vi "Teleop.vi"(10 "Match Info":T1={"Autonomous Elapsed Seconds"=0.0, "TeleOp Elapsed Seconds"=0.0, "Disabled Elapsed Seconds"=0.0, "Visited Autonomous"=FALSE, "Visited TeleOp"=FALSE, "Visited Disabled"=FALSE, "Autonomous Settings"={"Autonomous Style"=enum."Independent", "VI Refnum"=refnum}}, 11 "Call Context":T2) -> ()   [LabVIEW 2013]
doc: "This VI is called for each TeleOp packet received from the DS where the robot is not disabled. It is often used to read from the joysticks and update I/O or to update setpoints for timed control loops. It should complete and return within 20 milliseconds or it may miss DS packets."
uses:
  <vilib>/Rock Robotics/WPI/DriverStation/WPI_DriverStationDerivedRobotMode.ctl
  <vilib>/Rock Robotics/WPI/DriverStation/WPI_DriverStationMatch Info.ctl
  Robot Global Data.vi
  <vilib>/Rock Robotics/WPI/Joystick/WPI_JoystickGetSetRefNum.vi
  <vilib>/Rock Robotics/WPI/RobotDrive/WPI_RobotDriveGetSetRefNum.vi
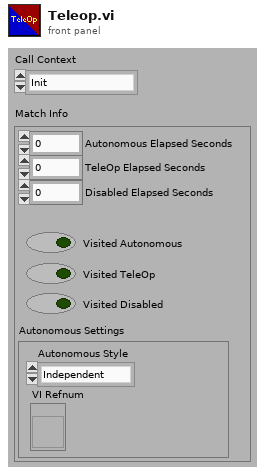
[diagram p1: front panel]
types:
  T1 = typedef "WPI_DriverStationMatch Info.ctl" = cluster{"Autonomous Elapsed Seconds":dbl, "TeleOp Elapsed Seconds":dbl, "Disabled Elapsed Seconds":dbl, "Visited Autonomous":bool, "Visited TeleOp":bool, "Visited Disabled":bool, "Autonomous Settings":cluster{"Autonomous Style":enum16{"Iterative", "Independent"}, "VI Refnum":refnum<vi>}}
  T2 = typedef "WPI_DriverStationDerivedRobotMode.ctl" = enum16{"Init", "Execute", "Stop"}
  T3 = typedef "WPI_JoystickDevRef.ctl" = cluster{"Device":T4}
  T4 = typedef "WPI_JoystickDeviceEnum.ctl" = enum16{"USB 1", "USB 2", "USB 3", "USB 4", "Kinect 1", "Kinect 2"}
  T5 = cluster{"axis 1 (x)":dbl, "axis 2 (y)":dbl, "axis 3 (throttle)":dbl, "axis 4":dbl, "axis 5":dbl, "axis 6":dbl}
  T6 = typedef "WPI_RobotDriveDevRef.ctl" = cluster{"DevStatus":errorcluster, "Motors[]":T7[], "Square Inputs":bool, "Max Output":dbl, "Isochronous":bool}
  T7 = typedef "WPI_MotorControlDeviceRef.ctl" = cluster{"DeviceStatus":errorcluster, "Type":enum16{"PWM", "CAN"}, "PWM":cluster{"Digital Module":T8, "PWM Channel":T9, "DeadBand":T10}, "CAN":cluster{"Device Number":u8, "Control Mode":T11, "Semaphore":T12, "Max Vout":dbl}, "Invert":bool, "TransformRef":T13, "InvTransformRef":T13}
  T8 = typedef "FPGA_TypedefDigitalModule.ctl" = enum16{"Digital Module 1", "Digital Module 2"}
  T9 = typedef "FPGA_DIOPWMChannel.ctl" = enum8{"PWM 1", "PWM 2", "PWM 3", "PWM 4", "PWM 5", "PWM 6", "PWM 7", "PWM 8", "PWM 9", "PWM 10", "Invalid"}
  T10 = typedef "WPI_PWMDeadband.ctl" = cluster{"Name":string, "maxPositivePwm":i32, "minPositivePwm":i32, "centerPwm":i32, "maxNegativePwm":i32, "minNegativePwm":i32, "angularRange":u16}
  T11 = typedef "WPI_CANJaguar_ControlMode.ctl" = enum8{"Percent VBus", "Current", "Speed", "Position", "Voltage"}
  T12 = typedef "Semaphore RefNum" = refnum<k1>
  T13 = typedef "WPI_PWMTransform_ConPane.ctl" = refnum<vi>
  T14 = enum16{"ToPos2", "ToPos1", "Fire", "Wait", "ESTOP", "Reset", "ToLowPower", "ToHighPower"}
  T15 = typedef "WPI_JoystickButtonState.ctl" = cluster{"Button 1":bool, "Button 2":bool, "Button 3":bool, "Button 4":bool, "Button 5":bool, "Button 6":bool, "Button 7":bool, "Button 8":bool, "Button 9":bool, "Button 10":bool, "Button 11":bool, "Button 12":bool}
  T16 = typedef "WPI_DigitalInputDevRef.ctl" = cluster{"DevStatus":errorcluster, "DIO Channel":T17, "Digital Module":T8}
  T17 = typedef "FPGA_DIOChannel.ctl" = enum8{"DIO 1", "DIO 2", "DIO 3", "DIO 4", "DIO 5", "DIO 6", "DIO 7", "DIO 8", "DIO 9", "DIO 10", "DIO 11", "DIO 12", "DIO 13", "DIO 14", "Invalid"}
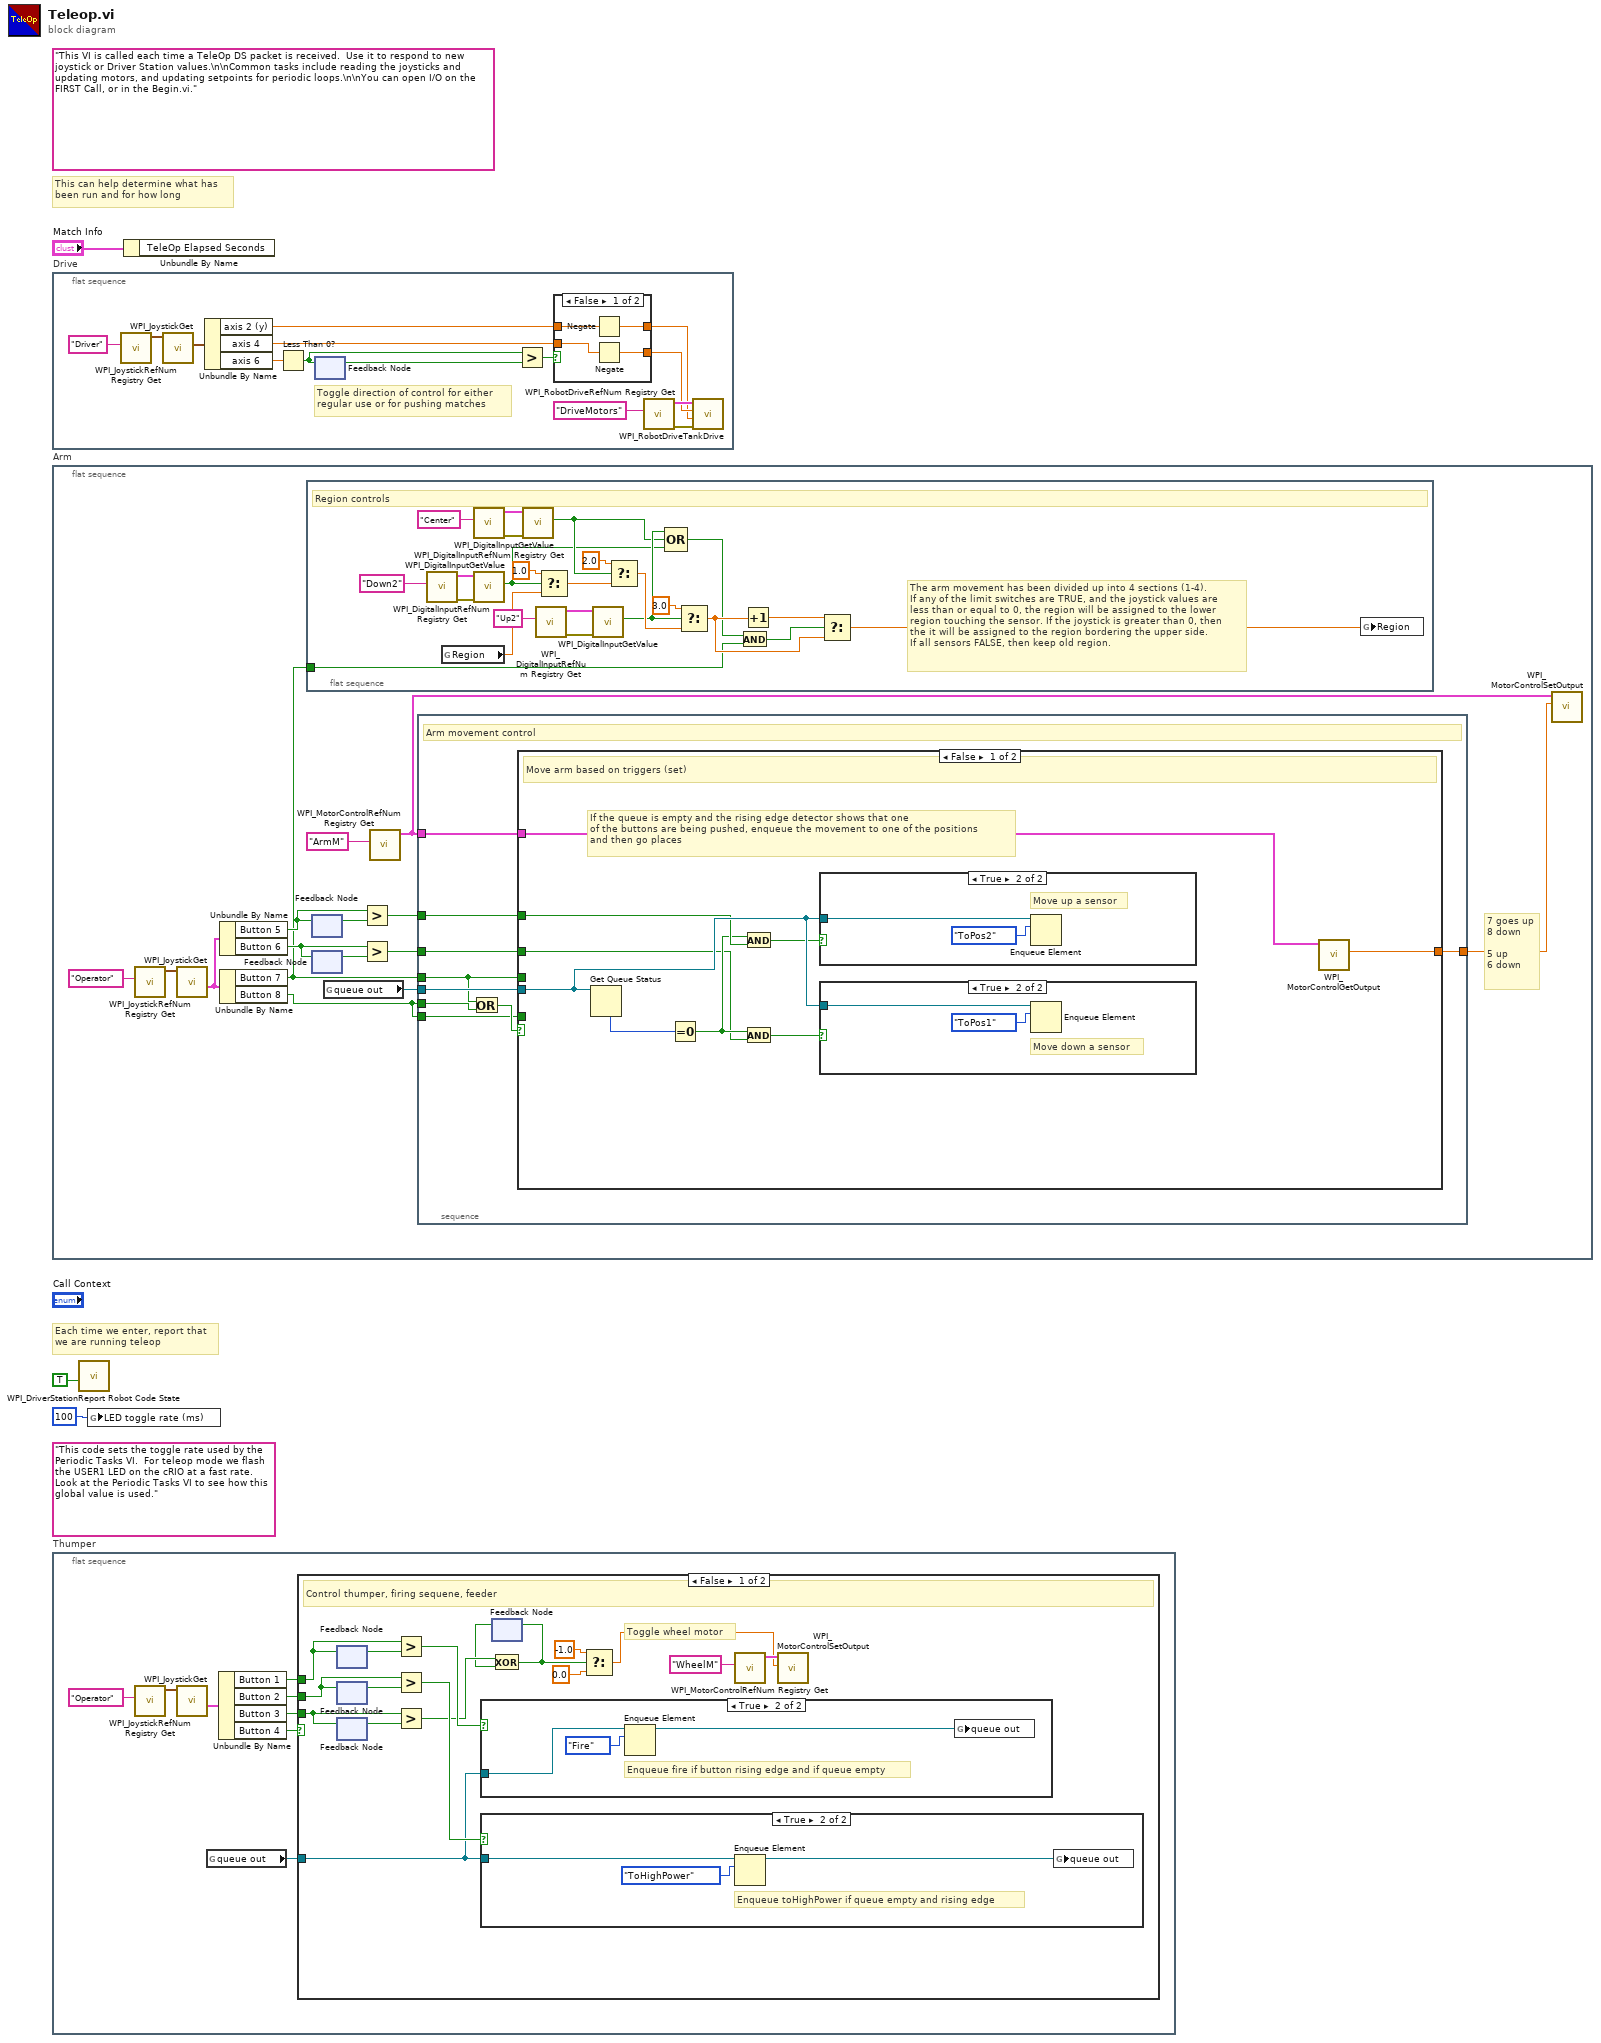
[diagram p0: block diagram]
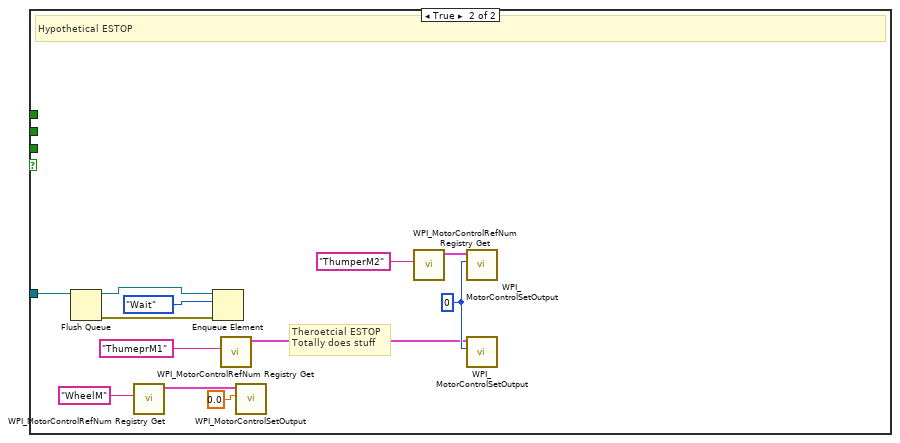
[diagram p4: hidden frame]
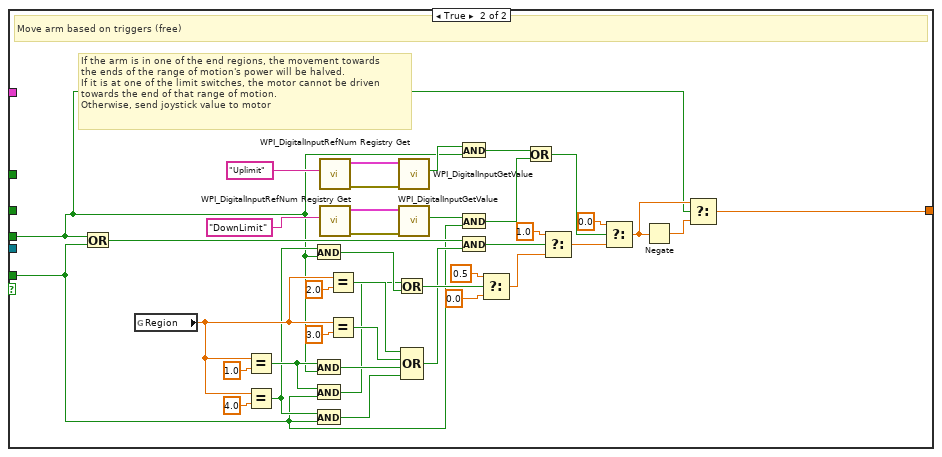
[diagram p7: hidden frame]
diagram:
  (unwired) "This code sets the toggle rate used by the Periodic Tasks VI.  For teleop mode we flash the USER1 LED on the cRIO at a fast rate.  Look at the Periodic Tasks VI to see how this global value is used."
  (unwired) "This VI is called each time a TeleOp DS packet is received.  Use it to respond to new joystick or Driver Station values.\n\nCommon tasks include reading the joysticks and updating motors, and updating setpoints for periodic loops.\n\nYou can open I/O on the FIRST Call, or in the Begin.vi."
  # "Each time we enter, report that\nwe are running teleop"
  # "This can help determine what has\nbeen run and for how long"
  n1 = flat-sequence "Drive" {
    frame #0 {
      # "Toggle direction of control for either\nregular use or for pushing matches"
      n2 = call <vilib>:"WPI_JoystickRefNum Registry Get.vi"("refnum name"="Driver") -> ("JoystickDevRef"=w15:T3)  [unwired: 1 in, 9 out]
      n3 = call <vilib>:"WPI_JoystickGet.vi"("JoystickDevRef"=w15) -> ("Axes"=w14:T5)  [unwired: 1 in, 5 out]
      n4 = Unbundle By Name(w14) -> ("axis 2 (y)"=w10:dbl, "axis 4"=w9:dbl, "axis 6"=w5:dbl)
      n5 = Less Than 0?(x=w5) -> (x < 0?=w7:bool)
      n6 = feedback-in #1(w7) -> ()
      n7 = feedback #1() -> (w6:bool)  [unwired: 1 in]
      n8 = Greater?(x=w7, y=w6) -> (0:w4:bool)
      n9 = case shown="False" w4 {
        tunnel: [w19 w23] -> w11
        tunnel: w10 -> [w21 w23]
        tunnel: w9 -> [w20 w22]
        tunnel: [w18 w22] -> w8
        frame False {
          n10 = Negate(x=w21) -> (-x=w18:dbl)
          n11 = Negate(x=w20) -> (-x=w19:dbl)
        }
        frame True {
        }
      }
      n12 = call <vilib>:"WPI_RobotDriveRefNum Registry Get.vi"("refnum name"="DriveMotors") -> ("error out"=w12:errorcluster, "RobotDriveDevRef"=w13:T6)  [unwired: 1 in, 8 out]
      n13 = call <vilib>:"WPI_RobotDriveTankDrive.vi"("error in (no error)"=w12, "Right axis value"=w8, "Left axis value"=w11, "RobotDriveDevRef"=w13) -> ()  [unwired: 5 in, 3 out]
    }
  }
  n14 = flat-sequence "Arm" {
    frame #0 {
      # "7 goes up\n8 down\n\n5 up\n6 down"
      n15 = call <vilib>:"WPI_JoystickRefNum Registry Get.vi"("refnum name"="Operator") -> ("JoystickDevRef"=w36:T3)  [unwired: 1 in, 9 out]
      n16 = call <vilib>:"WPI_JoystickGet.vi"("JoystickDevRef"=w36) -> ("Buttons"=w26:T15)  [unwired: 1 in, 5 out]
      n17 = Unbundle By Name(w26) -> ("Button 5"=w33:bool, "Button 6"=w31:bool)
      n18 = Unbundle By Name(w26) -> ("Button 7"=w25:bool, "Button 8"=w24:bool)
      n19 = flat-sequence {
        tunnel: w25 -> [w42]
        frame #0 {
          # "The arm movement has been divided up into 4 sections (1-4).\nIf any of the limit switches are TRUE, and the joystick values are\nless than or equal to 0, the region will be assigned to the lower\nregion touching the sensor. If the joystick is greater than 0, then\nthe it will be assigned to the region bordering the upper side.\nIf all sensors FALSE, then keep old region."
          # "Region controls"
          n20 = call <vilib>:"WPI_DigitalInputRefNum Registry Get.vi"("refnum name"="Down2") -> ("error out"=w61:errorcluster, "DigitalInputDevRef"=w62:T16)  [unwired: 9 in]
          n21 = global read "Robot Global Data.vi" "Region"() -> (w45:dbl)
          n22 = call <vilib>:"WPI_DigitalInputRefNum Registry Get.vi"("refnum name"="Center") -> ("error out"=w58:errorcluster, "DigitalInputDevRef"=w59:T16)  [unwired: 9 in]
          n23 = call <vilib>:"WPI_DigitalInputGetValue.vi"("error in (no error)"=w61, "DigitalInputDevRef"=w62) -> ("Value"=w39:bool)  [unwired: 7 in, 2 out]
          n24 = call <vilib>:"WPI_DigitalInputGetValue.vi"("error in (no error)"=w58, "DigitalInputDevRef"=w59) -> ("Value"=w40:bool)  [unwired: 7 in, 2 out]
          n25 = call <vilib>:"WPI_DigitalInputRefNum Registry Get.vi"("refnum name"="Up2") -> ("error out"=w55:errorcluster, "DigitalInputDevRef"=w56:T16)  [unwired: 9 in]
          n26 = Select(t=1.0, s=w39, f=w45) -> (s? t:f=w50:dbl)
          n27 = call <vilib>:"WPI_DigitalInputGetValue.vi"("error in (no error)"=w55, "DigitalInputDevRef"=w56) -> ("Value"=w41:bool)  [unwired: 7 in, 2 out]
          n28 = Select(t=2.0, s=w40, f=w50) -> (s? t:f=w49:dbl)
          n29 = Compound Arithmetic op=OR(w41, w40, w39) -> (w44:bool)
          n30 = Select(t=3.0, s=w41, f=w49) -> (s? t:f=w48:dbl)
          n31 = And(x=w44, y=w42) -> (x .and. y?=w43:bool)
          n32 = Increment(x=w48) -> (x+1=w47:dbl)
          n33 = Select(t=w47, s=w43, f=w48) -> (s? t:f=w46:dbl)
          n34 = global write "Robot Global Data.vi" "Region"(w46) -> ()
        }
      }
      n35 = feedback-in #2(w33) -> ()
      n36 = feedback #2() -> (w34:bool)  [unwired: 1 in]
      n37 = feedback #3() -> (w32:bool)  [unwired: 1 in]
      n38 = feedback-in #3(w31) -> ()
      n39 = global read "Robot Global Data.vi" "queue out"() -> (w28:refnum<queue>)
      n40 = Greater?(x=w33, y=w34) -> (0:w29:bool)
      n41 = Greater?(x=w31, y=w32) -> (0:w30:bool)
      n42 = call <vilib>:"WPI_MotorControlRefNum Registry Get.vi"("refnum name"="ArmM") -> ("MotorControlDevRef"=w27:T7)  [unwired: 9 in, 1 out]
      n43 = stacked-sequence {
        tunnel: [w71] -> w35
        tunnel: w25 -> [w65]
        tunnel: w30 -> [w70]
        tunnel: w29 -> [w69]
        tunnel: w28 -> [w68]
        tunnel: w27 -> [w67]
        tunnel: w24 -> [w64]
        tunnel: w24 -> [w63]
        frame #0 {
          # "Arm movement control"
          n44 = Or(x=w65, y=w64) -> (x .or. y?=w66:bool)
          n45 = case shown="False" w66 {
            tunnel: [w80 w92] -> w71
            tunnel: w65 -> [_ w86]
            tunnel: w70 -> [w75 _]
            tunnel: w69 -> [w77 _]
            tunnel: w68 -> [w78 _]
            tunnel: w67 -> [w72 _]
            tunnel: w63 -> [_ w85]
            frame False {
              # "If the queue is empty and the rising edge detector shows that one\nof the buttons are being pushed, enqueue the movement to one of the positions\nand then go places"
              # "Move arm based on triggers (set)"
              n46 = Get Queue Status(queue=w78) -> (# elements in queue=w79:i32)  [unwired: 2 in, 7 out]
              n47 = Equal To 0?(x=w79) -> (x = 0?=w76:bool)
              n48 = And(x=w76, y=w77) -> (x .and. y?=w74:bool)
              n49 = And(x=w76, y=w75) -> (x .and. y?=w73:bool)
              n50 = case shown="True" w74 {
                tunnel: w78 -> [_ w83]
                frame False {
                }
                frame True {
                  # "Move up a sensor"
                  n51 = Enqueue Element(queue=w83, element=T14."ToPos2") -> ()  [unwired: 2 in, 3 out]
                }
              }
              n52 = case shown="True" w73 {
                tunnel: w78 -> [_ w81]
                frame False {
                }
                frame True {
                  # "Move down a sensor"
                  n53 = Enqueue Element(queue=w81, element=T14."ToPos1") -> ()  [unwired: 2 in, 3 out]
                }
              }
              n54 = call <vilib>:"WPI_MotorControlGetOutput.vi"("MotorControlDevRef"=w72) -> ("Output"=w80:dbl)  [unwired: 8 in, 2 out]
            }
            frame True {
              # "If the arm is in one of the end regions, the movement towards \nthe ends of the range of motion's power will be halved.\nIf it is at one of the limit switches, the motor cannot be driven\ntowards the end of that range of motion.\nOtherwise, send joystick value to motor"
              # "Move arm based on triggers (free)"
              n55 = Or(x=w86, y=w85) -> (x .or. y?=w87:bool)
              n56 = global read "Robot Global Data.vi" "Region"() -> (w110:dbl)
              n57 = Equal?(x=w110, y=1.0) -> (x = y?=w105:bool)
              n58 = Equal?(x=w110, y=4.0) -> (x = y?=w104:bool)
              n59 = And(x=w104, y=w86) -> (x .and. y?=w107:bool)
              n60 = And(x=w105, y=w86) -> (x .and. y?=w113:bool)
              n61 = And(x=w105, y=w85) -> (x .and. y?=w106:bool)
              n62 = And(x=w104, y=w85) -> (x .and. y?=w112:bool)
              n63 = call <vilib>:"WPI_DigitalInputRefNum Registry Get.vi"("refnum name"="Uplimit") -> ("error out"=w120:errorcluster, "DigitalInputDevRef"=w121:T16)  [unwired: 9 in]
              n64 = call <vilib>:"WPI_DigitalInputRefNum Registry Get.vi"("refnum name"="DownLimit") -> ("error out"=w122:errorcluster, "DigitalInputDevRef"=w123:T16)  [unwired: 9 in]
              n65 = Equal?(x=w110, y=2.0) -> (x = y?=w117:bool)
              n66 = Equal?(x=w110, y=3.0) -> (x = y?=w115:bool)
              n67 = Or(x=w106, y=w107) -> (x .or. y?=w103:bool)
              n68 = call <vilib>:"WPI_DigitalInputGetValue.vi"("error in (no error)"=w120, "DigitalInputDevRef"=w121) -> ("Value"=w100:bool)  [unwired: 7 in, 2 out]
              n69 = call <vilib>:"WPI_DigitalInputGetValue.vi"("error in (no error)"=w122, "DigitalInputDevRef"=w123) -> ("Value"=w96:bool)  [unwired: 7 in, 2 out]
              n70 = Compound Arithmetic op=OR(w117, w115, w113, w112) -> (w88:bool)
              n71 = And(x=w100, y=w86) -> (x .and. y?=w99:bool)
              n72 = And(x=w96, y=w85) -> (x .and. y?=w98:bool)
              n73 = And(x=w87, y=w88) -> (x .and. y?=w89:bool)
              n74 = Select(t=0.5, s=w103, f=0.0) -> (s? t:f=w101:dbl)
              n75 = Or(x=w99, y=w98) -> (x .or. y?=w97:bool)
              n76 = Select(t=1.0, s=w89, f=w101) -> (s? t:f=w93:dbl)
              n77 = Select(t=0.0, s=w97, f=w93) -> (s? t:f=w90:dbl)
              n78 = Negate(x=w90) -> (-x=w91:dbl)
              n79 = Select(t=w90, s=w86, f=w91) -> (s? t:f=w92:dbl)
            }
          }
        }
      }
      n80 = call <vilib>:"WPI_MotorControlSetOutput.vi"("Output"=w35, "MotorControlDevRef"=w27) -> ()  [unwired: 7 in, 3 out]
    }
  }
  n81 = flat-sequence "Thumper" {
    frame #0 {
      n82 = call <vilib>:"WPI_JoystickRefNum Registry Get.vi"("refnum name"="Operator") -> ("JoystickDevRef"=w131:T3)  [unwired: 9 in, 1 out]
      n83 = call <vilib>:"WPI_JoystickGet.vi"("JoystickDevRef"=w131) -> ("Buttons"=w130:T15)  [unwired: 4 in, 2 out]
      n84 = global read "Robot Global Data.vi" "queue out"() -> (w124:refnum<queue>)
      n85 = Unbundle By Name(w130) -> ("Button 1"=w127:bool, "Button 2"=w128:bool, "Button 3"=w129:bool, "Button 4"=w125:bool)
      n86 = case shown="False" w125 {
        tunnel: w129 -> [w148 _]
        tunnel: w128 -> [w143 _]
        tunnel: w127 -> [w142 _]
        tunnel: w124 -> [w132 w160]
        frame False {
          # "Toggle wheel motor"
          # "Control thumper, firing sequene, feeder"
          n87 = feedback #4() -> (w141:bool)  [unwired: 1 in]
          n88 = feedback-in #4(w142) -> ()
          n89 = feedback #5() -> (w140:bool)  [unwired: 1 in]
          n90 = feedback-in #5(w143) -> ()
          n91 = feedback #6() -> (w147:bool)  [unwired: 1 in]
          n92 = feedback-in #6(w148) -> ()
          n93 = Greater?(x=w142, y=w141) -> (0:w138:bool)
          n94 = Greater?(x=w143, y=w140) -> (0:w139:bool)
          n95 = Greater?(x=w148, y=w147) -> (0:w137:bool)
          n96 = case shown="True" w138 {
            tunnel: w132 -> [_ w152]
            frame False {
            }
            frame True {
              # "Enqueue fire if button rising edge and if queue empty"
              n97 = Enqueue Element(queue=w152, element=T14."Fire") -> (queue out=w154:refnum<queue>)  [unwired: 2 in, 2 out]
              n98 = global write "Robot Global Data.vi" "queue out"(w154) -> ()
            }
          }
          n99 = case shown="True" w139 {
            tunnel: w132 -> [_ w151]
            frame False {
            }
            frame True {
              # "Enqueue toHighPower if queue empty and rising edge"
              n100 = Enqueue Element(queue=w151, element=T14."ToHighPower") -> (queue out=w150:refnum<queue>)  [unwired: 2 in, 2 out]
              n101 = global write "Robot Global Data.vi" "queue out"(w150) -> ()
            }
          }
          n102 = feedback #7() -> (w134:bool)  [unwired: 1 in]
          n103 = Exclusive Or(1:w134, 2:w137) -> (0:w133:bool)
          n104 = feedback-in #7(w133) -> ()
          n105 = Select(t=-1.0, s=w133, f=0.0) -> (s? t:f=w144:dbl)
          n106 = call <vilib>:"WPI_MotorControlRefNum Registry Get.vi"("refnum name"="WheelM") -> ("MotorControlDevRef"=w145:T7)  [unwired: 9 in, 1 out]
          n107 = call <vilib>:"WPI_MotorControlSetOutput.vi"("Output"=w144, "MotorControlDevRef"=w145) -> ()  [unwired: 7 in, 3 out]
        }
        frame True {
          w159 = 0
          # "Theroetcial ESTOP\nTotally does stuff"
          # "Hypothetical ESTOP"
          n108 = Flush Queue(queue=w160) -> (queue out=w161:refnum<queue>, error out=w162:errorcluster)  [unwired: 1 in, 1 out]
          n109 = call <vilib>:"WPI_MotorControlRefNum Registry Get.vi"("refnum name"="WheelM") -> ("MotorControlDevRef"=w165:T7)  [unwired: 9 in, 1 out]
          n110 = Enqueue Element(queue=w161, element=T14."Wait", error in (no error)=w162) -> ()  [unwired: 1 in, 3 out]
          n111 = call <vilib>:"WPI_MotorControlRefNum Registry Get.vi"("refnum name"="ThumeprM1") -> ("MotorControlDevRef"=w157:T7)  [unwired: 9 in, 1 out]
          n112 = call <vilib>:"WPI_MotorControlSetOutput.vi"("Output"=0.0 ("t"), "MotorControlDevRef"=w165) -> ()  [unwired: 7 in, 3 out]
          n113 = call <vilib>:"WPI_MotorControlRefNum Registry Get.vi"("refnum name"="ThumperM2") -> ("MotorControlDevRef"=w158:T7)  [unwired: 9 in, 1 out]
          n114 = call <vilib>:"WPI_MotorControlSetOutput.vi"("Output"=w159, "MotorControlDevRef"=w158) -> ()  [unwired: 7 in, 3 out]
          n115 = call <vilib>:"WPI_MotorControlSetOutput.vi"("Output"=w159, "MotorControlDevRef"=w157) -> ()  [unwired: 7 in, 3 out]
        }
      }
    }
  }
  n116 = call <vilib>:"WPI_DriverStationReport Robot Code State.vi"("TeleOp"=TRUE ("Autonomous")) -> ()  [unwired: 10 in, 1 out]
  n117 = global write "Robot Global Data.vi" "LED toggle rate (ms)"(u32 100 ("LED ms toggle rate")) -> ()
  n118 = Unbundle By Name("Match Info") -> ()  [unwired: 1 out]
